vi "OnseShotPulse.vi"(11 "Input":bool) -> (3 "Output":bool)   [LabVIEW 2016]
doc: "Outputs true on the first iteration the input goes true, then is false until the input goes false and true again"
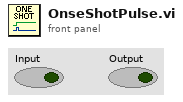
[diagram p1: front panel]
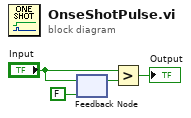
[diagram p0: block diagram]
diagram:
  n1 = feedback #1(FALSE) -> (w1:bool)
  n2 = feedback-in #1("Input") -> ()
  n3 = Greater?(x="Input", y=w1) -> (0:→"Output":bool)
